vi "Leave Process Loop.vi"(8 "error in (no error)":errorcluster, 11 "Process In":refnum<class "Debug View.lvclass">) -> (0 "error out":errorcluster, 3 "Process Out":refnum<class "Debug View.lvclass">)   [LabVIEW 2020]
doc: "Clears the in process loop flag. This VI should be called if a branch of the process instance is sent out of the process loop to avoid undefined behavior."
uses:
  Debug View.lvclass
  Debug View.lvclass/Debug View.ctl
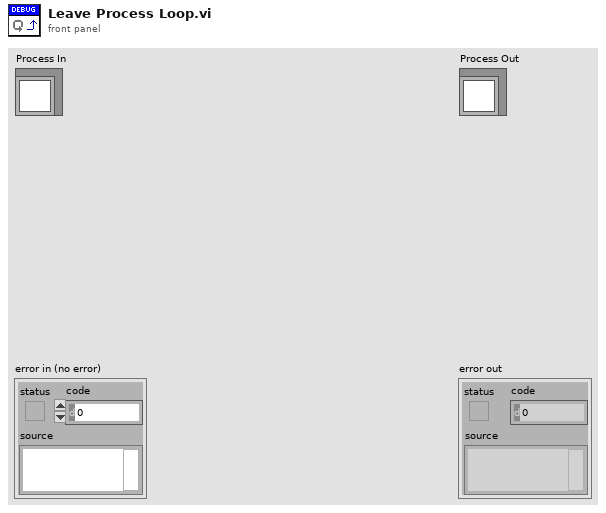
[diagram p1: front panel]
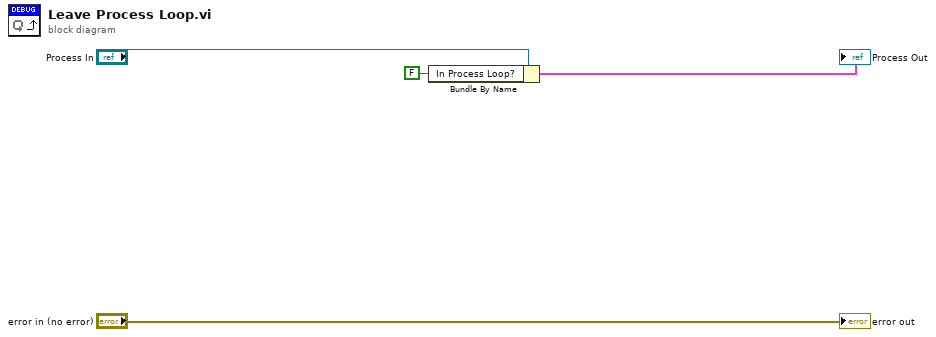
[diagram p0: block diagram]
diagram:
  n1 = Bundle By Name(cluster="Process In", "In Process Loop?"=FALSE) -> (→"Process Out":cluster{})
  "error out" <- "error in (no error)"
